vi "MaxiGauge_Main_Panel.vi"(8 "input cluster":T1) -> ()   [LabVIEW 2019]
uses:
  cluster_ref_MaxiGauge.ctl
panel:
  out "Last Updated":timestamp format="%<%Y-%m-%d %H:%M:%S>T"
  out "GAUGE  Status: (Channel 1, 2, 3, 4, 5, 6, )":string
  in  "Channel 6":enum16{"NO CHANGE", "OFF", "ON"}(ring)
  in  "Channel 5":enum16{"NO CHANGE", "OFF", "ON"}(ring)
  in  "Channel 4":enum16{"NO CHANGE", "OFF", "ON"}(ring)
  in  "Channel 3":enum16{"NO CHANGE", "OFF", "ON"}(ring)
  in  "Channel 2":enum16{"NO CHANGE", "OFF", "ON"}(ring)
  in  "Channel 1":enum16{"NO CHANGE", "OFF", "ON"}(ring)
  in  "Gauge On/Off/Status":bool
  out "Sensor Type: (Channel 1, 2, 3, 4, 5, 6, )":string
  in  "Get Pressure sensor type":bool
  in  "Maxi_visa":refnum<visa-resource-name>="COM8"
  in  "Measurement Rate (ms)":i32
  out "Channel 6":string
  out "Channel 5":string
  out "Channel 4":string
  out "Channel 3":string
  out "Channel 2":string
  out "Channel 1":string
  # "Gauge On/Off/Status"
  # "Pressure Value\n(Torr)"
  # "Gauge status:\n1 = OFF\n2 = ON"
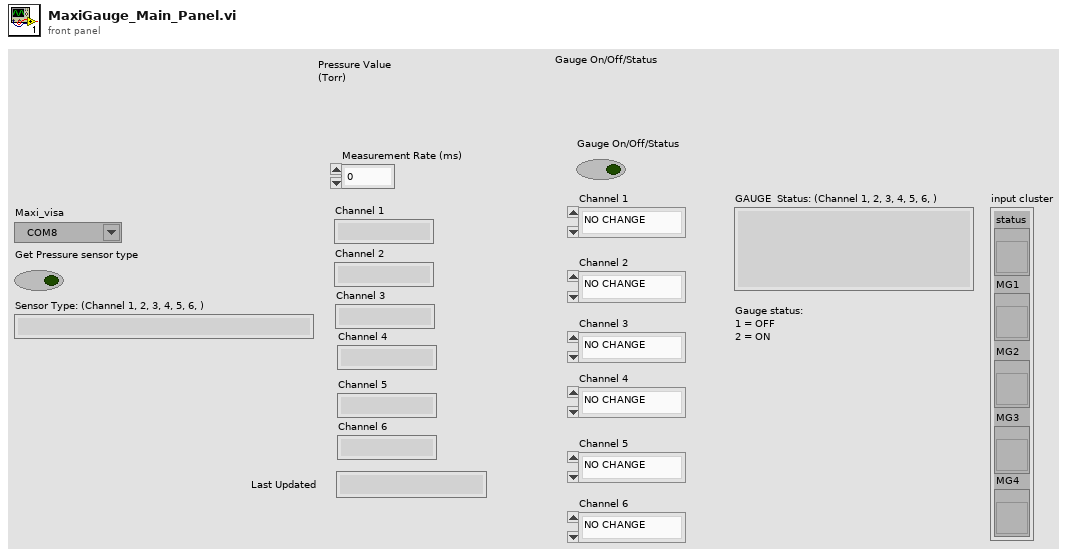
[diagram p1: front panel]
types:
  T1 = typedef "cluster_ref_MaxiGauge.ctl" = cluster{"status":refnum<vi>, "MG1":refnum<vi>, "MG2":refnum<vi>, "MG3":refnum<vi>, "MG4":refnum<vi>}
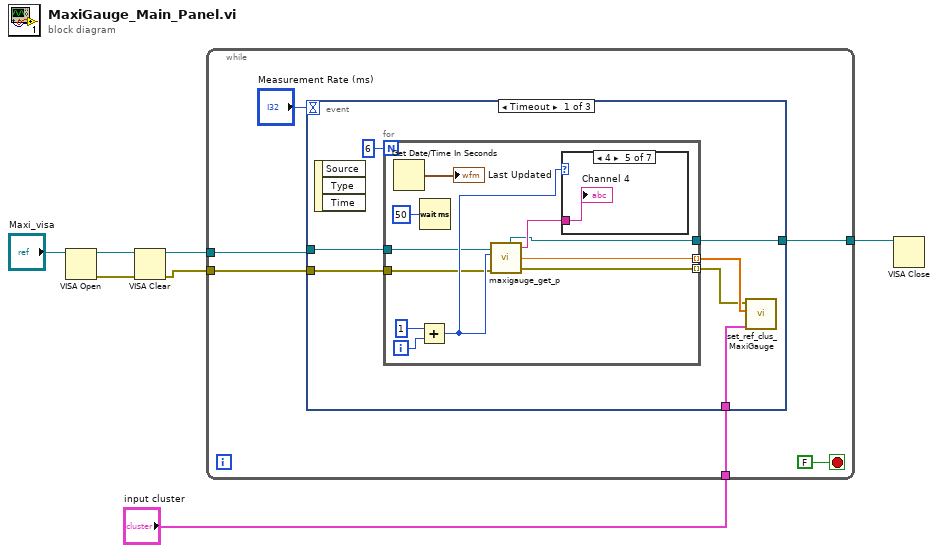
[diagram p0: block diagram]
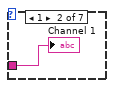
[diagram p3: hidden frame]
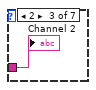
[diagram p4: hidden frame]
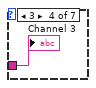
[diagram p5: hidden frame]
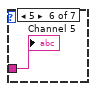
[diagram p6: hidden frame]
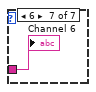
[diagram p7: hidden frame]
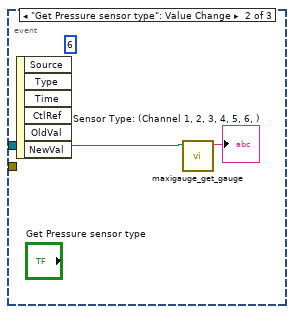
[diagram p8: hidden frame]
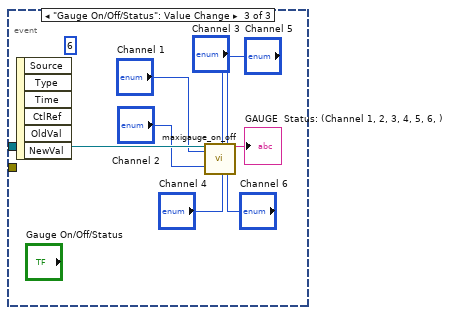
[diagram p9: hidden frame]
diagram:
  n1 = VISA Open(VISA resource name="Maxi_visa") -> (VISA resource name=w6:refnum<visa-resource-name>, error out=w2:errorcluster)  [unwired: 4 in]
  n2 = VISA Clear(VISA resource name=w6, error in (no error)=w2) -> (VISA resource name out=w3:refnum<visa-resource-name>, error out=w1:errorcluster)
  n3 = while {
    tunnel: "input cluster" -> [w11]
    tunnel: w3 -> [w10]
    tunnel: [w9] -> w4
    tunnel: w1 -> [w8]
    stop <- FALSE stop-if-true
    n4 = event shown="[0] Timeout" {
      selector: _ -> [_ _ _]
      dyn-events: _ -> [_ _ _]
      timeout: "Measurement Rate (ms)" -> [_ _ _]
      tunnel: w10 -> [w19 w39 w47]
      tunnel: w11 -> [w18 _ _]
      tunnel: [w15 _ _] -> w9
      tunnel: w8 -> [w14 _ _]
      event Timeout {
        n5 = event-data() -> ()  [unwired: 1 in, 3 out]
        n6 = for {
          N: 6 -> [_]
          tunnel: w19 -> [w26]
          tunnel: [w24] -> w17 mode=indexing
          tunnel: [w23] -> w16 mode=indexing
          tunnel: [w22] -> w15
          tunnel: w14 -> [w21]
          i -> [w31]
          n7 = Get Date/Time In Seconds() -> (seconds since 1Jan1904=→"Last Updated":timestamp)
          n8 = Add(x=1, y=w31) -> (x+y=w28:i32)
          n9 = Wait (ms)(milliseconds to wait=u32 50) -> ()  [unwired: 1 out]
          n10 = call "maxigauge_get_p.vi"("err_in"=w21, 9:w28, "maxi_visa"=w26) -> ("err_out"=w23:errorcluster, "pressure"=w24:dbl, "Pressure (Torr)"=w27:string, "maxi_visa 2"=w22:refnum<visa-resource-name>)  [unwired: 4 in]
          n11 = case shown="4" w28 {
            tunnel: w27 -> [_ w32 w33 w34 w35 w36 w37]
            frame 0, Default {
            }
            frame 1 {
              "Channel 1" <- w32
            }
            frame 2 {
              "Channel 2" <- w33
            }
            frame 3 {
              "Channel 3" <- w34
            }
            frame 4 {
              "Channel 4" <- w35
            }
            frame 5 {
              "Channel 5" <- w36
            }
            frame 6 {
              "Channel 6" <- w37
            }
          }
        }
        n12 = call "set_ref_clus_MaxiGauge.vi"("input cluster"=w18, "value_array"=w17, "error_array"=w16) -> ()  [unwired: 9 in]
      }
      event "Get Pressure sensor type": Value Change {
        (unwired) 6
        n13 = event-data() -> ()  [unwired: 1 in, 6 out]
        n14 = call "maxigauge_get_gauge.vi"("maxi_visa"=w39) -> ("Gauge Type"=→"Sensor Type: (Channel 1, 2, 3, 4, 5, 6, )":string)  [unwired: 8 in, 1 out]
      }
      event "Gauge On/Off/Status": Value Change {
        (unwired) 6
        n15 = event-data() -> ()  [unwired: 1 in, 6 out]
        n16 = call "maxigauge_on_off.vi"("maxi_visa"=w47, "Channel 1"="Channel 1", "Channel 2"="Channel 2", "Channel 3"="Channel 3", "Channel 4"="Channel 4", "Channel 5"="Channel 5", "Channel 6"="Channel 6") -> ("GAUGE  Status"=→"GAUGE  Status: (Channel 1, 2, 3, 4, 5, 6, )":string)  [unwired: 11 in, 1 out]
      }
    }
  }
  n17 = VISA Close(VISA resource name=w4) -> ()  [unwired: 1 in, 1 out]
